vi "motorMoveVector-Old-Controllers.vi"(3 "Motor (XYZ)":string(combo)="X", 4 "Distance":sgl, 5 "Device in":refnum<k24>) -> (2 "Device out":refnum<k24>)   [LabVIEW 2014]
doc: "André Romero - 2017\nandretec@ifsc.usp.br"
uses:
  C:/UserLabs/Andre/LabView2014-32bits/kinesisTec/Kinesis/Thorlabs.MotionControl.TCube.DCServoCLI.dll
  Kinesis/Thorlabs.MotionControl.TCube.DCServoCLI.dll
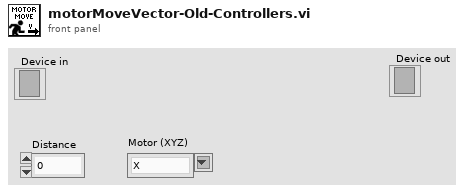
[diagram p1: front panel]
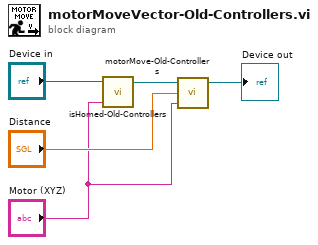
[diagram p0: block diagram]
diagram:
  n1 = call "isHomed-Old-Controllers.vi"("Motor (XYZ)"="Motor (XYZ)", "Device in"="Device in") -> ("Device out"=w4:refnum<k24>)  [unwired: 3 in]
  n2 = call "motorMove-Old-Controllers.vi"("Motor (XYZ)"="Motor (XYZ)", "position"="Distance", "Device in"=w4) -> ("Device out"=→"Device out":refnum<k24>)  [unwired: 2 in]
